vi "CV08_DAQmx_subvi.vi"(8 "error in":errorcluster, 9 "data in":waveform(dbl), 10 "AO channel":tag, 11 "AI channel":tag) -> (0 "error out":errorcluster, 2 "data out":waveform(dbl))   [LabVIEW 2023]
uses:
  <vilib>/DAQmx/write.llb/DAQmx Write (Analog Wfm 1Chan NSamp).vi
  <vilib>/DAQmx/read.llb/DAQmx Read (Analog Wfm 1Chan NSamp).vi
  <vilib>/DAQmx/create/channels.llb/DAQmx Create Channel (AO-Voltage-Basic).vi
  <vilib>/DAQmx/configure/timing.llb/DAQmx Timing (Sample Clock).vi
  <vilib>/DAQmx/miscellaneous.llb/DAQmx Fill In Error Info.vi
  <vilib>/DAQmx/create/channels.llb/DAQmx Create Channel (AI-Voltage-Basic).vi
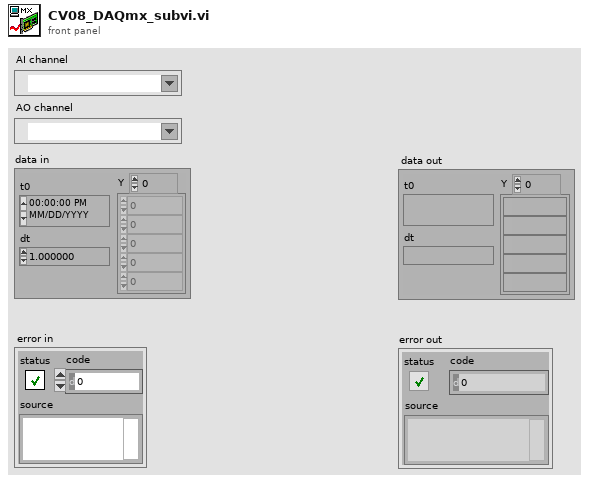
[diagram p1: front panel]
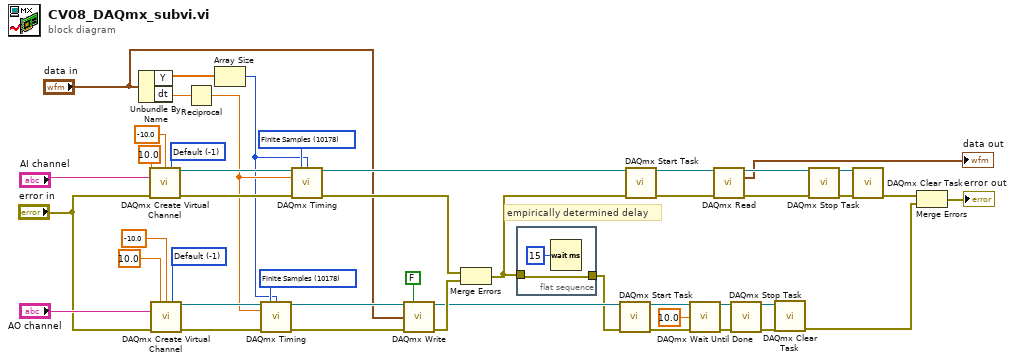
[diagram p0: block diagram]
diagram:
  w8 = -1 items=["Default"=-1, "RSE"=10083, "Differential"=10106, "Pseudodifferential"=12529] ("output terminal configuration")
  w29 = 10178 items=["Finite Samples"=10178, "Continuous Samples"=10123, "Hardware Timed Single Point"=12522] ("sample mode")
  w41 = -1 items=["Default"=-1, "RSE"=10083, "NRSE"=10078, "Differential"=10106, "Pseudodifferential"=12529] ("input terminal configuration")
  w44 = 10178 items=["Finite Samples"=10178, "Continuous Samples"=10123, "Hardware Timed Single Point"=12522] ("sample mode")
  # "empirically determined delay"
  n1 = Unbundle By Name("data in") -> ("Y"=w27:dbl[], "dt"=w28:dbl)
  n2 = call-poly <vilib>:"DAQmx Create Virtual Channel.vi"("maximum value"=10.0, "minimum value"=-10.0, "input terminal configuration"=w41, "physical channels"="AI channel", "error in"="error in") -> ("task out"=w40:refnum<k21>, "error out"=w39:errorcluster)  [unwired: 9 in]
  n3 = call-poly <vilib>:"DAQmx Create Virtual Channel.vi"("maximum value"=10.0, "minimum value"=-10.0, "output terminal configuration"=w8, "physical channels"="AO channel", "error in"="error in") -> ("task out"=w46:refnum<k21>, "error out"=w45:errorcluster)  [unwired: 9 in]
  n4 = Reciprocal(x=w28) -> (1/x=w5:dbl)
  n5 = Array Size(array=w27) -> (size(s)=w4:i32)
  n6 = call-poly <vilib>:"DAQmx Timing.vi"("task/channels in"=w46, "sample mode"=w44, "samples per channel"=w4, "rate"=w5, "error in"=w45) -> ("task out"=w26:refnum<k21>, "error out"=w12:errorcluster)  [unwired: 9 in]
  n7 = call-poly <vilib>:"DAQmx Timing.vi"("task/channels in"=w40, "sample mode"=w29, "samples per channel"=w4, "rate"=w5, "error in"=w39) -> ("task out"=w25:refnum<k21>, "error out"=w24:errorcluster)  [unwired: 9 in]
  n8 = call-poly <vilib>:"DAQmx Write.vi"("task/channels in"=w26, "auto start"=FALSE, "data"="data in", "error in"=w12) -> ("task out"=w21:refnum<k21>, "error out"=w22:errorcluster)  [unwired: 9 in, 1 out]
  n9 = Merge Errors(w24, w22) -> (w14:errorcluster)
  n10 = flat-sequence {
    tunnel: w14 -> [w47]
    tunnel: [w47] -> w13
    frame #0 {
      n11 = Wait (ms)(milliseconds to wait=u32 15) -> ()  [unwired: 1 out]
    }
  }
  n12 = call <vilib>:"DAQmx Start Task.vi"("task/channels in"=w21, "error in"=w13) -> ("task out"=w19:refnum<k21>, "error out"=w20:errorcluster)  [unwired: 12 in]
  n13 = call <vilib>:"DAQmx Start Task.vi"("task/channels in"=w25, "error in"=w14) -> ("task out"=w38:refnum<k21>, "error out"=w37:errorcluster)  [unwired: 12 in]
  n14 = call <vilib>:"DAQmx Wait Until Done.vi"("task/channels in"=w19, "timeout (sec)"=10.0, "error in"=w20) -> ("task out"=w16:refnum<k21>, "error out"=w17:errorcluster)  [unwired: 11 in]
  n15 = call-poly <vilib>:"DAQmx Read.vi"("task/channels in"=w38, "error in"=w37) -> ("task out"=w36:refnum<k21>, "data"=→"data out":waveform(dbl), "error out"=w35:errorcluster)  [unwired: 11 in]
  n16 = call <vilib>:"DAQmx Stop Task.vi"("task/channels in"=w16, "error in"=w17) -> ("task out"=w42:refnum<k21>, "error out"=w43:errorcluster)  [unwired: 12 in]
  n17 = call <vilib>:"DAQmx Clear Task.vi"("task in"=w42, "error in"=w43) -> ("error out"=w31:errorcluster)  [unwired: 13 in]
  n18 = call <vilib>:"DAQmx Stop Task.vi"("task/channels in"=w36, "error in"=w35) -> ("task out"=w34:refnum<k21>, "error out"=w33:errorcluster)  [unwired: 12 in]
  n19 = call <vilib>:"DAQmx Clear Task.vi"("task in"=w34, "error in"=w33) -> ("error out"=w32:errorcluster)  [unwired: 13 in]
  n20 = Merge Errors(w32, w31) -> (→"error out":errorcluster)
